vi "Save JPEG File.vi"(0 "Image In":T1, 2 "Color Palette In":cluster{"Red":u8, "Green":u8, "Blue":u8}[](array[cluster]), 11 "Error in (no error)":errorcluster, 13 "JPEG File Path":path) -> (4 "Image Out(dup)":T1, 15 "Error out":errorcluster)   [LabVIEW 2021]
uses:
  <resource>/objmgr/IMAQImage.rc
  <vilib>/vision/Image Controls.llb/IMAQ Image.ctl
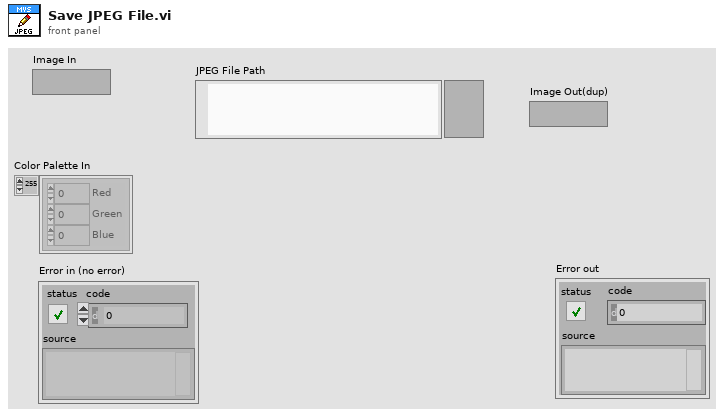
[diagram p1: front panel]
types:
  T1 = typedef "IMAQ Image.ctl" = refnum<image>
  T2 = typedef "imagedata.ctl" = cluster{"image type":i32, "image depth":i32, "image":u8[], "mask":u8[], "colors":u32[], "Rectangle":cluster{"left":i16, "top":i16, "right":i16, "bottom":i16}}
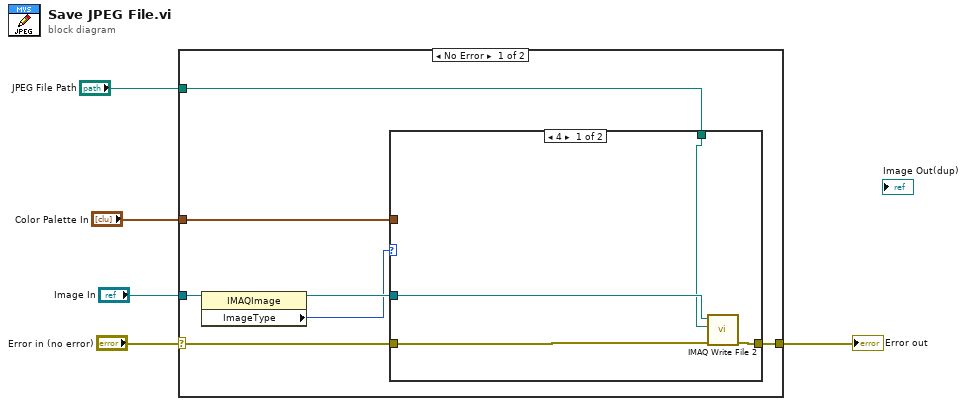
[diagram p0: block diagram]
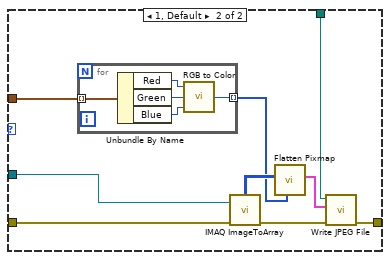
[diagram p2: hidden frame]
diagram:
  n1 = case shown="No Error" "Error in (no error)" {
    selector: "Error in (no error)" -> [w9 w31]
    tunnel: "Color Palette In" -> [w12 _]
    tunnel: "Image In" -> [w8 _]
    tunnel: "JPEG File Path" -> [w11 _]
    tunnel: [w10 w31] -> w2
    frame No Error {
      n2 = property class="IMAQImage"(reference=w8) -> (reference out=w7:T1, "ImageType"=w6:u32)  [unwired: 1 in, 1 out]
      n3 = case shown="4" w6 {
        tunnel: w12 -> [_ w22]
        tunnel: w11 -> [w13 w20]
        tunnel: [w15 w19] -> w10
        tunnel: w9 -> [w16 w18]
        tunnel: w7 -> [w14 w17]
        frame 4 {
          n4 = call-poly "IMAQ Write File 2"("error in (no error)"=w16, "File Path"=w13, "Image"=w14) -> ("error out"=w15:errorcluster)  [unwired: 7 in, 1 out]
        }
        frame 1, Default {
          n5 = for {
            tunnel: w22 -> [w30] mode=indexing
            tunnel: [w26] -> w23 mode=indexing
            n6 = Unbundle By Name(w30) -> ("Red"=w29:u8, "Green"=w28:u8, "Blue"=w27:u8)
            n7 = call <vilib>:"RGB to Color.vi"("B"=w27, "G"=w28, "R"=w29) -> ("Color"=w26:u32)
          }
          n8 = call "IMAQ ImageToArray"("error in (no error)"=w18, "Image"=w17) -> ("error out"=w21:errorcluster, "Image Pixels (U8)"=w25:u8[][])  [unwired: 2 in, 3 out]
          n9 = call <vilib>:"Flatten Pixmap.vi"("colors"=w23, "8-bit pixmap"=w25) -> ("image data"=w24:T2)  [unwired: 9 in]
          n10 = call <vilib>:"Write JPEG File.vi"("error in (no error)"=w21, "image data"=w24, "path to JPEG file"=w20) -> ("error out"=w19:errorcluster)  [unwired: 7 in, 1 out]
        }
      }
    }
    frame Error {
    }
  }
  "Error out" <- w2
